vi "Acquire Module Semaphore.vi"(8 "error in":errorcluster) -> (0 "error out":errorcluster)   [LabVIEW 2020, in "Singleton Module.lvlib"]
doc: "Acquire the module semaphore.\n_____\nBased on DQMH Project Template 6.1.0.93."
uses:
  Singleton Module.lvlib
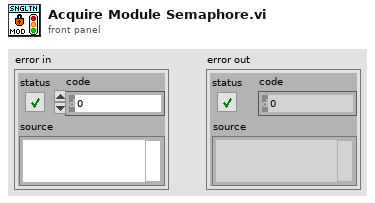
[diagram p1: front panel]
types:
  T1 = typedef "Semaphore RefNum" = refnum<k1>
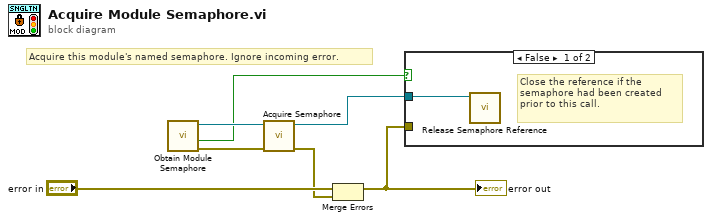
[diagram p0: block diagram]
diagram:
  # "Acquire this module's named semaphore. Ignore incoming error."
  n1 = call "Obtain Module Semaphore.vi"() -> ("error out"=w5:errorcluster, "created new?"=w2:bool, "semaphore"=w3:T1)  [unwired: 9 in]
  n2 = call <vilib>:"Acquire Semaphore.vi"("error in (no error)"=w5, "semaphore"=w3) -> ("error out"=w6:errorcluster, "semaphore out"=w1:T1)  [unwired: 3 in, 1 out]
  n3 = Merge Errors("error in", w6) -> (w4:errorcluster)
  "error out" <- w4
  n4 = case shown="False" w2 {
    tunnel: w1 -> [w8 _]
    tunnel: w4 -> [_ _]
    frame False {
      # "Close the reference if the semaphore had been created prior to this call."
      n5 = call <vilib>:"Release Semaphore Reference.vi"("semaphore"=w8) -> ()  [unwired: 9 in, 2 out]
    }
    frame True {
    }
  }
